vi "RotationDirectionSet.vi"(3 "error in (no error)":errorcluster, 4 "Counterclockwise":bool caption="Clockwise", 5 "VISA resource name":refnum<visa-resource-name>) -> (0 "error out":errorcluster, 1 "Command not accepted":bool, 2 "VISA resource name out":refnum<visa-resource-name>)   [LabVIEW 2017, in "Spectral Products CM110.lvlib"]
uses:
  Spectral Products CM110.lvlib
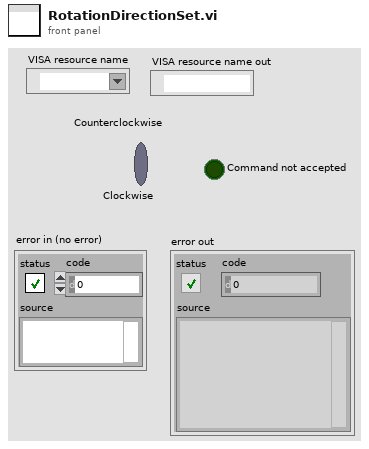
[diagram p1: front panel]
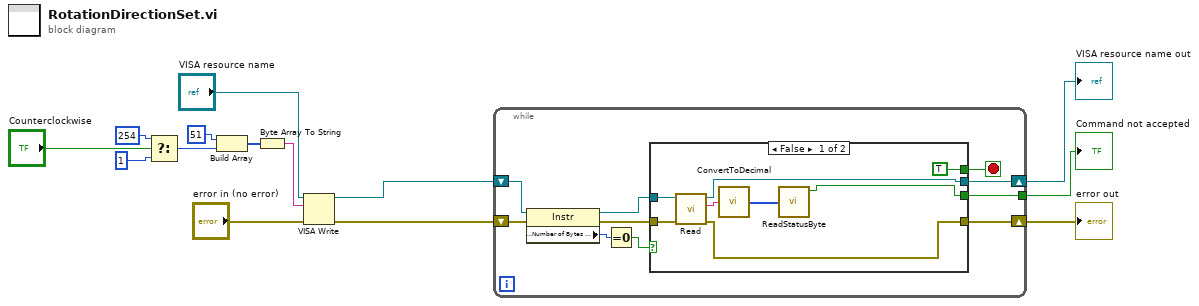
[diagram p0: block diagram]
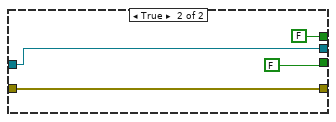
[diagram p2: hidden frame]
diagram:
  n1 = Select(t=u8 254, s="Counterclockwise", f=u8 1) -> (s? t:f=w6:u8)
  n2 = Build Array(u8 51, w6) -> (w11:u8[])
  n3 = Byte Array To String(unsigned byte array=w11) -> (string=w10:string)
  n4 = VISA Write(VISA resource name="VISA resource name", write buffer=w10, error in (no error)="error in (no error)") -> (VISA resource name out=w2:refnum<visa-resource-name>, error out=w1:errorcluster)  [unwired: 1 out]
  n5 = while {
    shift-right: [w17] -> w3
    shift-left: w2 -> [w24]
    shift-right: [w16] -> w5
    shift-left: w1 -> [w23]
    tunnel: [w15] -> w4
    stop <- w22 stop-if-true
    n6 = property class="Instr"(reference=w24, error in=w23) -> (reference out=w21:refnum<visa-resource-name>, error out=w20:errorcluster, "Serial Settings:Number of Bytes at Serial Port"=w19:u32)
    n7 = Equal To 0?(x=w19) -> (x = 0?=w18:bool)
    n8 = case shown="False" w18 {
      tunnel: [TRUE FALSE] -> w22
      tunnel: w21 -> [w32 w35]
      tunnel: w20 -> [w31 w34]
      tunnel: [w28 w35] -> w17
      tunnel: [w25 w34] -> w16
      tunnel: [w26 FALSE] -> w15
      frame False {
        n9 = call "Read.vi"("error in (no error)"=w31, "VISA Refnum in"=w32) -> ("error out"=w25:errorcluster, "read buffer"=w30:string, "VISA Refnum out"=w28:refnum<visa-resource-name>)  [unwired: 6 in, 1 out]
        n10 = call "ConvertToDecimal.vi"("read buffer"=w30) -> ("unsigned byte array"=w27:u8[])
        n11 = call "ReadStatusByte.vi"("unsigned byte array"=w27) -> ("Command not accepted"=w26:bool)  [unwired: 4 in, 5 out]
      }
      frame True {
      }
    }
  }
  "VISA resource name out" <- w3
  "error out" <- w5
  "Command not accepted" <- w4
